vi "5.4-6.7.4-How Server.vi"() -> ()   [LabVIEW 2010]
doc: "Creates a named service and listens on the first available port. Whenever a client connects to the service, it responds with a message containing joystick data. The VI can be stopped using the STOP button."
uses:
  6-OCU Neurons/6.0-Super Heart Beat.ctl
  6-OCU Neurons/6.4-How Reporting Typedef.ctl
  5.7-UDP/5.7 LabVIEW Errors.ctl
  5.0-Global.vi
panel:
  out "Status":errorcluster
  out "6.4 How Reporting":T1
  out "Super Heart Beat":T2
  in  "error in 2":errorcluster={"status"=TRUE, "code"=0, "source"=""}
  out "error out":errorcluster
  in  "stop":bool
  out "Probably a hello string":string
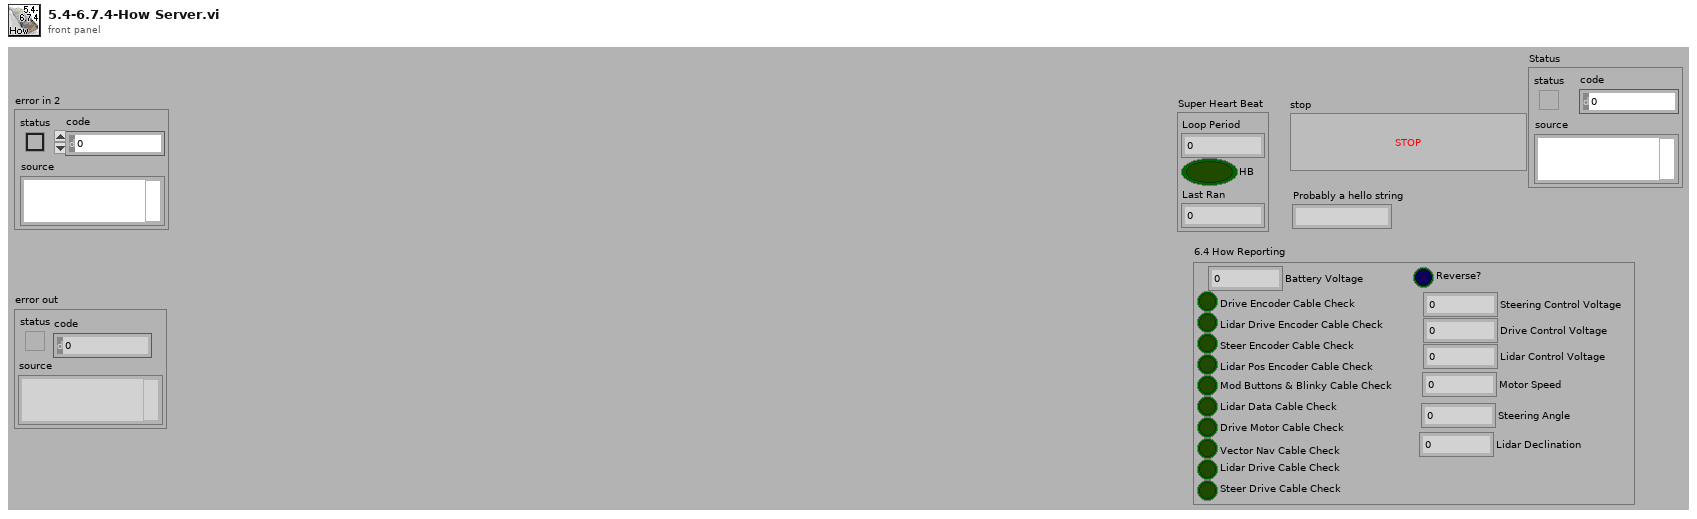
[diagram p1: front panel]
types:
  T1 = typedef "6.4-How Reporting Typedef.ctl" = cluster{"Motor Speed":i32, "Lidar Declination":i32, "Steering Angle":i32, "Battery Voltage":dbl, "Drive Encoder Cable Check":bool, "Lidar Drive Encoder Cable Check":bool, "Steer Encoder Cable Check":bool, "Lidar Pos Encoder Cable Check":bool, "Mod Buttons & Blinky Cable Check":bool, "Lidar Data Cable Check":bool, "Drive Motor Cable Check":bool, "Vector Nav Cable Check":bool, "Lidar Drive Cable Check":bool, "Steer Drive Cable Check":bool, "Reverse?":bool, "Steering Control Voltage":dbl, "Drive Control Voltage":dbl, "Lidar Control Voltage":dbl}
  T2 = typedef "6.0-Super Heart Beat.ctl" = cluster{"Loop Period":u32, "HB":bool, "Last Ran":u32}
  T3 = typedef "5.7 LabVIEW Errors.ctl" = i32
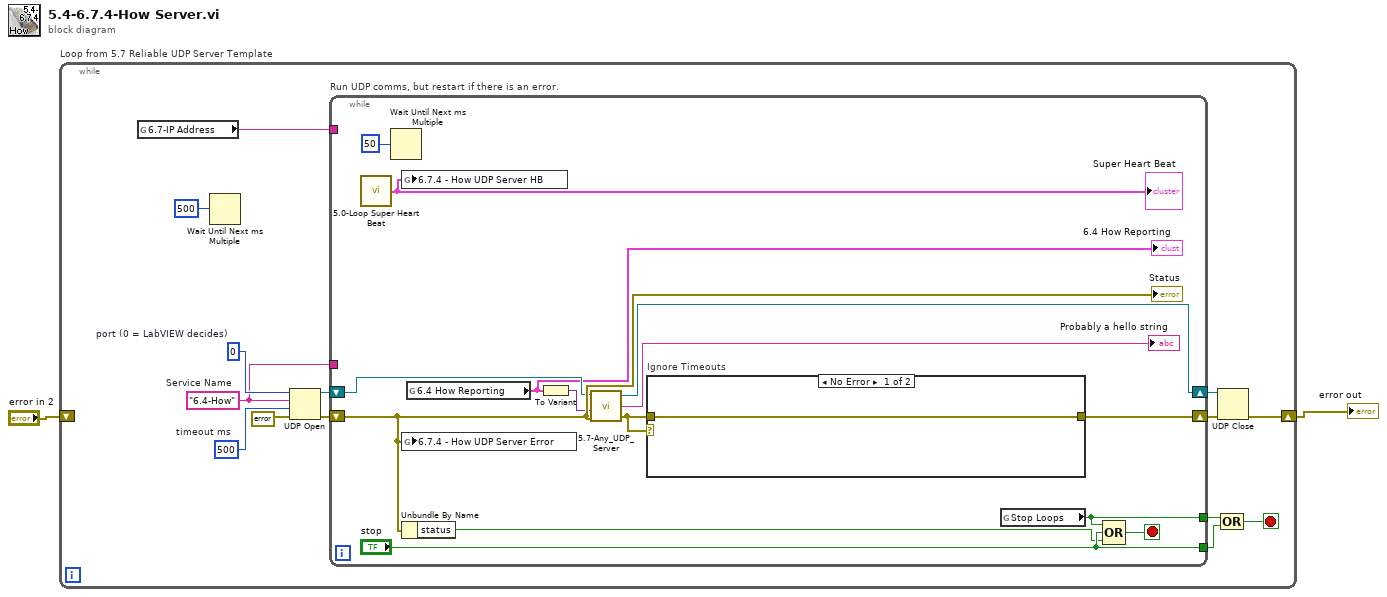
[diagram p0: block diagram]
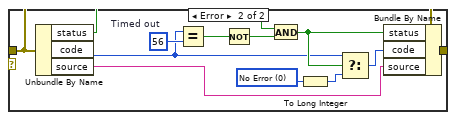
[diagram p2: hidden frame]
diagram:
  n1 = while "Loop from 5.7 Reliable UDP Server Template" {
    shift-right: [w9] -> w1
    shift-left: "error in 2" -> [_]
    stop <- w14 stop-if-true
    w6 = 500  # timeout ms
    w8 = u16 0  # port (0 = LabVIEW decides)
    w7 = "6.4-How"  # Service Name
    n2 = global read "5.0-Global.vi" "6.7-IP Address"() -> (w5:string)
    n3 = Wait Until Next ms Multiple(millisecond multiple=u32 500) -> ()  [unwired: 1 out]
    n4 = UDP Open(8:errorcluster {"status"=FALSE, "code"=0, "source"=""} ("error in (no error)"), 9:w6, 10:w7, 11:w8) -> (port=w13:refnum<k16>, 0:w11:errorcluster)  [unwired: 1 in, 1 out]
    n5 = while "Run UDP comms, but restart if there is an error." {
      tunnel: w7 -> [_]
      tunnel: w5 -> [_]
      tunnel: [w28] -> w16
      tunnel: ["stop"] -> w15
      shift-right: [w21] -> w12
      shift-left: w13 -> [w22]
      shift-right: [w25] -> w10
      shift-left: w11 -> [w24]
      stop <- w30 stop-if-true
      n6 = call "5.0-Loop Super Heart Beat.vi"() -> ("Super Heart Beat"=w17:T2)
      "Super Heart Beat" <- w17
      n7 = Wait Until Next ms Multiple(millisecond multiple=u32 50) -> ()  [unwired: 1 out]
      n8 = global write "5.0-Global.vi" "6.7.4 - How UDP Server HB"(w17) -> ()
      n9 = global write "5.0-Global.vi" "6.7.4 - How UDP Server Error"(w24) -> ()
      n10 = Unbundle By Name(w24) -> ("status"=w26:bool)
      n11 = global read "5.0-Global.vi" "6.4 How Reporting"() -> (w18:T1)
      "6.4 How Reporting" <- w18
      n12 = To Variant(anything=w18) -> (Variant=w20:variant)
      n13 = call "5.7-Any_UDP_Server.vi"("error In"=w24, "Data in"=w20, "Connection ID"=w22) -> ("warning out"=w23:errorcluster, "data out"=→"Probably a hello string":string, "Connection ID out"=w21:refnum<k16>)  [unwired: 1 in]
      n14 = case "Ignore Timeouts" shown="No Error" w23 {
        tunnel: w23 -> [w31 w43]
        tunnel: [w31 w42] -> w25
        frame No Error {
        }
        frame Error {
          w33 = T3 0 items=["No Error", "Argument Error", "Memory Full", "Out of Zone", "End of File", "File Already Open", "Generic File IO Error", "File Not Found", "File Permission Error", "Disk Full", "Duplicate Path", "Too Many Files Open", "Not Enabled", "Resource File Not Found", "Cannot Add Resource", "Resource Not Found", "Image Not Found", "Image Memory Error", "Pen Does Not Exist", "Config Bad Type", "Config Token Not Found", "Config Parse Error", "Config Memory Error", "Bad External Code Format", "Bad External Code Offset", "External Code Not Present", "Null Window", "Destroy Window Mixup", "Null Menu", "Print Aborted", "Bad Print Record", "Print Driver Error", "Windows Error During Print", "Memory Error During Print", "Print Dialog Error", "Generic Print Error", "Invalid Device Refnum", "Device Not Found", "Device Parameter Error", "Device Unit Error", "Can't Open Device", "Device Call Aborted", "Generic Error", "Cancelled By User", "Object ID Too Low", "Object ID Too High", "Object Not In Heap", "Unknown Heap", "Bad DefProc ID", "DefProc Not In Table", "Message Out Of Range", "Null Method", "Unknown Message", "Manager Call Not Supported", "Bad address", "Connection In progress", "Connection timed out", "Connection is already in progress", "Network attribute not supported", "Network error", "Address in use", "System out of memory", "Connection aborted", "Connection refused", "Connection is not connected", "Connection is already connected", "Connection closed", "Initialize error (interapplication manager)", "Bad occurrence", "Wait on unbound occurrence handler", "Occurrence queue overflow", "Bad path", "Semaphore not signaled", "Unrecognized type (interapplication manager)"] ("1st Error to Convert")
          w41 = 56  # Timed out
          n15 = Unbundle By Name(w43) -> ("status"=w38:bool, "code"=w36:i32, "source"=w34:string)
          n16 = Equal?(x=w36, y=w41) -> (x = y?=w40:bool)
          n17 = Not(x=w40) -> (.not. x?=w39:bool)
          n18 = And(x=w38, y=w39) -> (x .and. y?=w37:bool)
          n19 = To Long Integer(number=w33) -> (32bit integer=w32:T3)
          n20 = Select(t=w36, s=w37, f=w32) -> (s? t:f=w35:T3)
          n21 = Bundle By Name(cluster=w43, "status"=w37, "code"=w35, "source"=w34) -> (w42:errorcluster)
        }
      }
      n22 = global read "5.0-Global.vi" "Stop Loops"() -> (w28:bool)
      n23 = Compound Arithmetic op=OR(w28, "stop", w26) -> (w30:bool)
      "Status" <- w24
    }
    n24 = UDP Close(connection ID=w12, 8:w10) -> (error out=w9:errorcluster)  [unwired: 1 out]
    n25 = Compound Arithmetic op=OR(w16, w15) -> (w14:bool)
  }
  "error out" <- w1
